vi "Temperature Sensing Test.vi"(8 "error in (no error)":errorcluster) -> (0 "error out":errorcluster, 1 "Temperature":dbl, 2 "VISA resource OUT":refnum<visa-resource-name>, 3 "Actual Result":string, 5 "Relative Humidity":dbl)   [LabVIEW 2022 SP3]
uses:
  <vilib>/Instr/_visa.llb/VISA Flush IO Buffer Mask.ctl
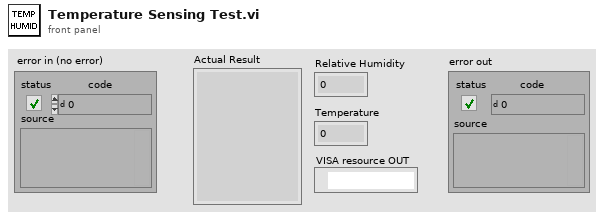
[diagram p1: front panel]
types:
  T1 = typedef "VISA Flush IO Buffer Mask.ctl" = u16
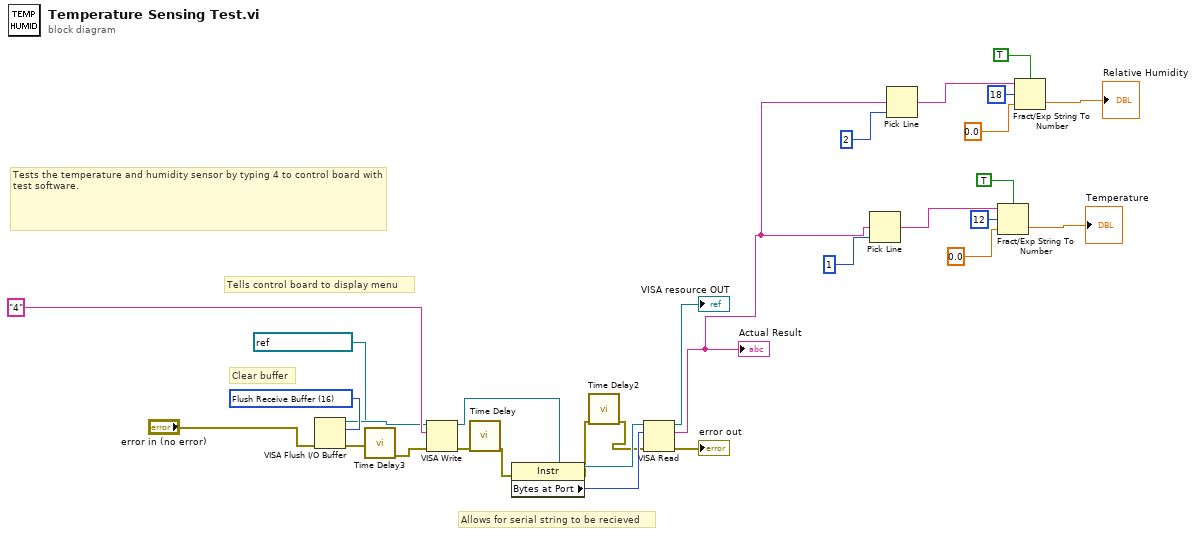
[diagram p0: block diagram]
diagram:
  w26 = T1 16 items=["Flush Receive Buffer"=16, "Write Transmit Buffer to Device"=32, "Flush Receive Buffer (No I/O)"=64, "Flush Transmit Buffer"=128] ("Mask")
  # "Tests the temperature and humidity sensor by typing 4 to control board with test software."
  # "Clear buffer"
  # "Allows for serial string to be recieved"
  # "Tells control board to display menu"
  n1 = VISA Flush I/O Buffer(VISA resource name=refnum<visa-resource-name> "ControlBoard", mask (16)=w26, error in (no error)="error in (no error)") -> (VISA resource name out=w24:refnum<visa-resource-name>, error out=w2:errorcluster)
  n2 = call "Time Delay3"("error in (no error)"=w2) -> ("error out"=w1:errorcluster)  [unwired: 10 in]
  n3 = VISA Write(VISA resource name=w24, write buffer="4", error in (no error)=w1) -> (VISA resource name out=w22:refnum<visa-resource-name>, error out=w25:errorcluster)  [unwired: 1 out]
  n4 = call "Time Delay"("error in (no error)"=w25) -> ("error out"=w23:errorcluster)  [unwired: 10 in]
  n5 = property class="Instr"(reference=w22, error in=w23) -> (reference out=w28:refnum<visa-resource-name>, error out=w17:errorcluster, "Bytes at Port"=w27:u32)
  n6 = call "Time Delay2"("error in (no error)"=w17) -> ("error out"=w16:errorcluster)  [unwired: 10 in]
  n7 = VISA Read(VISA resource name=w28, byte count=w27, error in (no error)=w16) -> (VISA resource name out=→"VISA resource OUT":refnum<visa-resource-name>, read buffer=w5:string, error out=→"error out":errorcluster)  [unwired: 1 out]
  "Actual Result" <- w5
  n8 = Pick Line(multi-line string=w5, line index=1) -> (output string=w14:string)  [unwired: 1 in]
  n9 = Pick Line(multi-line string=w5, line index=2) -> (output string=w9:string)  [unwired: 1 in]
  n10 = Fract/Exp String To Number(use system decimal point (T)=TRUE, string=w14, offset=12, default (0 dbl)=0.0 ("default (0 DBL)")) -> (number=→"Temperature":dbl)  [unwired: 1 out]
  n11 = Fract/Exp String To Number(use system decimal point (T)=TRUE, string=w9, offset=18, default (0 dbl)=0.0 ("default (0 DBL)")) -> (number=→"Relative Humidity":dbl)  [unwired: 1 out]
